vi "Calculate B Matrix.vi"(4 "threshold":dbl=0.0625 format="%#_13g", 6 "Tag ID":i32, 9 "Camera intrinsic matrix (K^-1)":dbl[][](array[numeric]), 10 "Homography H":T1) -> (0 "t (Translation Vector)":dbl[](array[numeric]), 1 "R Rotation Matrix (final)":T1 format="%#_6f", 2 "B Matrix":dbl[][](array[numeric]))   [LabVIEW 2025]
doc: "This VI calculates the full 6-DOF pose of an AprilTag relative to the camera. The algorithm converts the detected homography into camera coordinates using the intrinsic calibration matrix, then computes the tag translation vector and rotation matrix. A predictive filter is applied to the translation vector to reduce jitter and reject outlier measurements."
uses:
  <vilib>/Analysis/Matrix/Datatypes/RealMatrix.ctl
  <vilib>/Analysis/baseanly.llb/Real A x B.vi
  <vilib>/Analysis/baseanly.llb/Real Determinant.vi
  <vilib>/Analysis/7linalg.llb/Real SVD Decomposition.vi
  <vilib>/Analysis/NI_AALPro.lvlib
  <vilib>/Analysis/NI_AALBase.lvlib
  <vilib>/Analysis/Matrix/NI_Matrix.lvlib
panel:
  out "Matrix V":T1
  out "detR":dbl format="%.6f"
  out "detR_temp":dbl format="%.6f"
  out "R^tR":T1 format="%#.3f"
  out "v^t":T1 format="%#_6f"
  out "b1 lambda":dbl
  out "R Matrix":dbl[][](array[numeric])
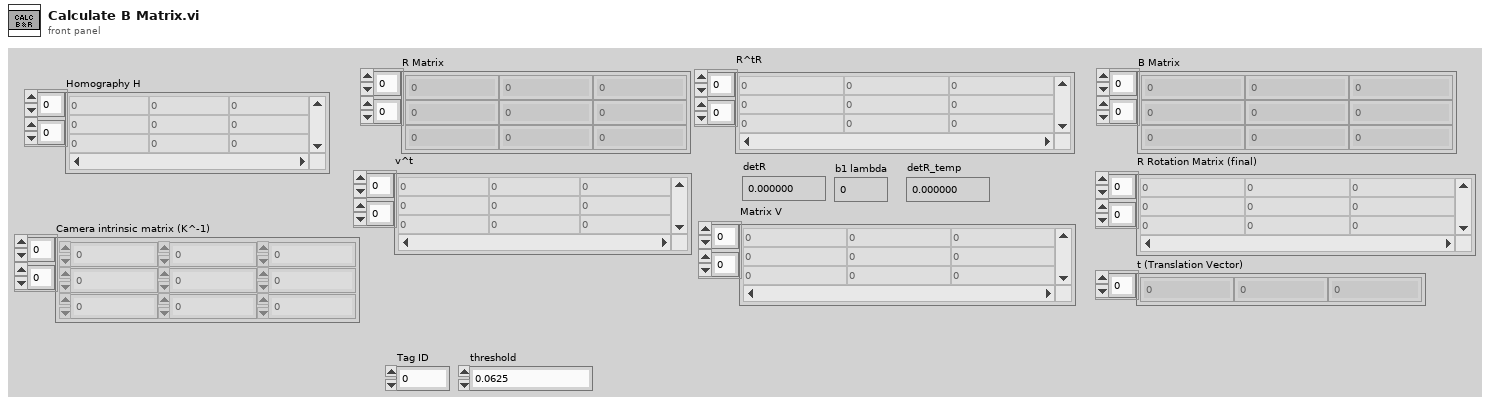
[diagram p1: front panel]
types:
  T1 = typedef "NI_Matrix.lvlib/RealMatrix.ctl" = dbl[][]
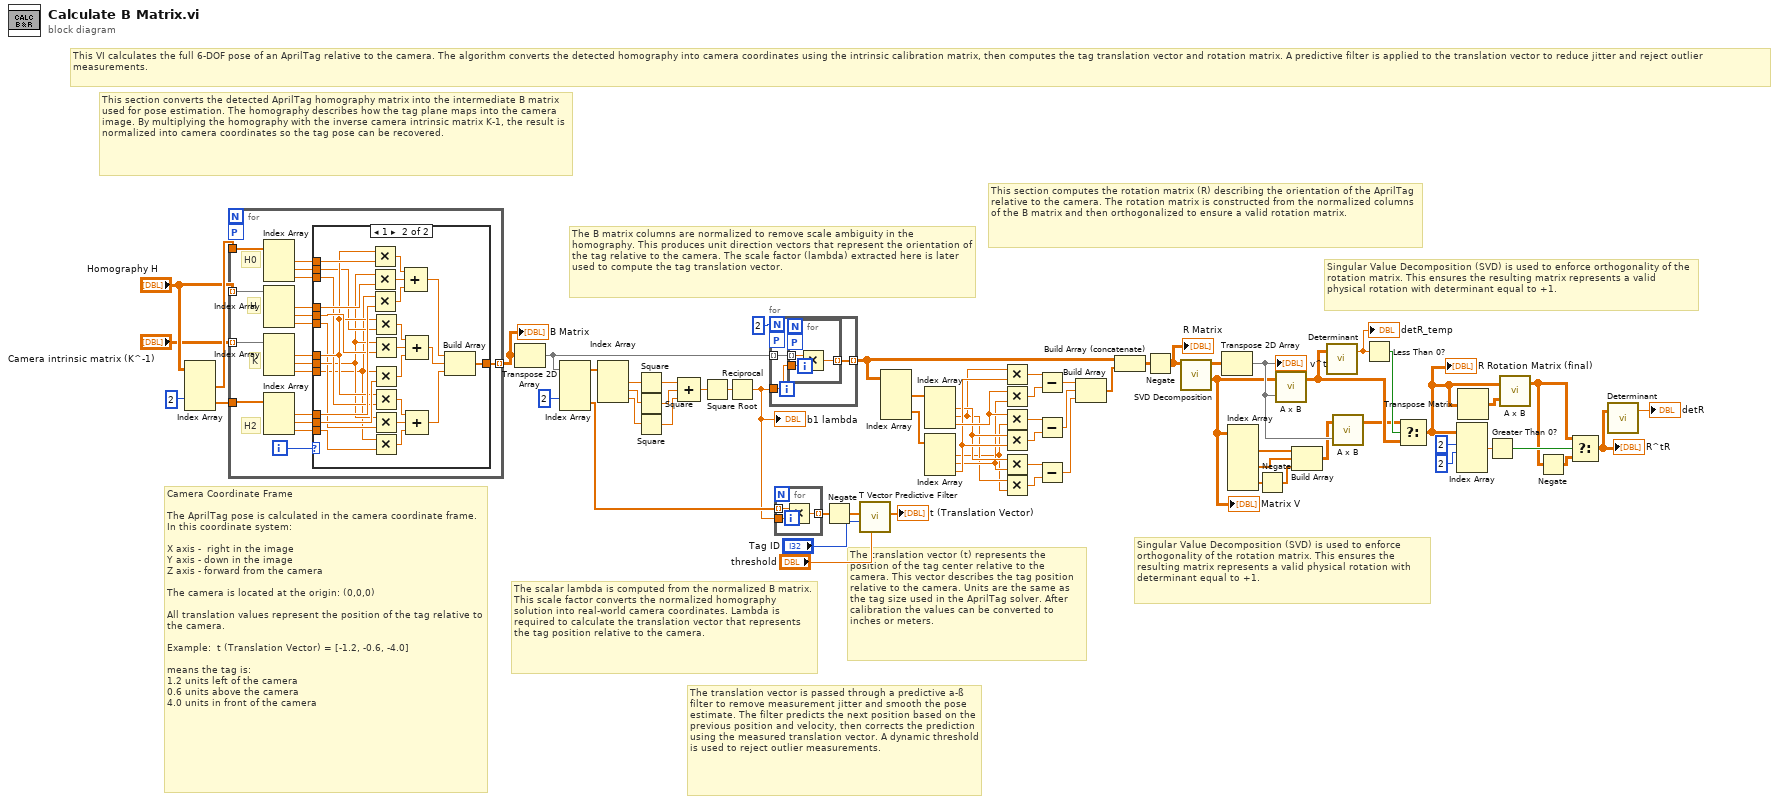
[diagram p0: block diagram]
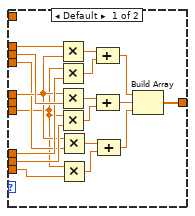
[diagram p2: hidden frame]
diagram:
  # "Camera Coordinate Frame\n\nThe AprilTag pose is calculated in the camera coordinate frame. In this coordinate system:\n\nX axis -  right in the image\nY axis - down in the image\nZ axis - forward from the camera\n\nThe camera is located at the origin: (0,0,0)\n\nAll translation values represent the position of the tag relative to the camera.\n\nExample:  t (Translation Vector) = [-1.2, -0.6, -4.0]\n\nmeans the tag is:\n1.2 units left of the camera\n0.6 units above the camera\n4.0 units in front of the camera"
  # "The translation vector (t) represents the position of the tag center relative to the camera. This vector describes the tag position relative to the camera. Units are the same as the tag size used in the AprilTag solver. After calibration the values can be converted to inches or meters."
  # "This VI calculates the full 6-DOF pose of an AprilTag relative to the camera. The algorithm converts the detected homography into camera coordinates using the intrinsic calibration matrix, then computes the tag translation vector and rotation matrix. A predictive filter is applied to the translation vector to reduce jitter and reject outlier measurements."
  # "Singular Value Decomposition (SVD) is used to enforce orthogonality of the rotation matrix. This ensures the resulting matrix represents a valid physical rotation with determinant equal to +1."
  # "Singular Value Decomposition (SVD) is used to enforce orthogonality of the rotation matrix. This ensures the resulting matrix represents a valid physical rotation with determinant equal to +1."
  # "This section computes the rotation matrix (R) describing the orientation of the AprilTag relative to the camera. The rotation matrix is constructed from the normalized columns of the B matrix and then orthogonalized to ensure a valid rotation matrix."
  # "The scalar lambda is computed from the normalized B matrix. This scale factor converts the normalized homography solution into real-world camera coordinates. Lambda is required to calculate the translation vector that represents the tag position relative to the camera."
  # "The B matrix columns are normalized to remove scale ambiguity in the homography. This produces unit direction vectors that represent the orientation of the tag relative to the camera. The scale factor (lambda) extracted here is later used to compute the tag translation vector."
  # "This section converts the detected AprilTag homography matrix into the intermediate B matrix used for pose estimation. The homography describes how the tag plane maps into the camera image. By multiplying the homography with the inverse camera intrinsic matrix K-1, the result is normalized into camera coordinates so the tag pose can be recovered."
  # "The translation vector is passed through a predictive a-ß filter to remove measurement jitter and smooth the pose estimate. The filter predicts the next position based on the previous position and velocity, then corrects the prediction using the measured translation vector. A dynamic threshold is used to reject outlier measurements."
  n1 = Index Array(array="Homography H", index (row) #2=2 ("index (row)")) -> (element #1=w68:dbl[], element #2=w67:dbl[])  [unwired: 3 in]
  n2 = for {
    tunnel: "Homography H" -> [w85] mode=indexing
    tunnel: "Camera intrinsic matrix (K^-1)" -> [w86] mode=indexing
    tunnel: w67 -> [w82]
    tunnel: [w75] -> w63 mode=indexing
    tunnel: w68 -> [w72]
    workers-P: _ -> [_]
    i -> [w74]
    # "H0"
    # "H2"
    # "K"
    # "H"
    n3 = Index Array(array=w72) -> (element #1=w71:dbl, element #2=w70:dbl, element #3=w69:dbl)  [unwired: 3 in]
    n4 = Index Array(array=w85) -> (element #1=w84:dbl, element #2=w83:dbl, element #3=w78:dbl)  [unwired: 3 in]
    n5 = Index Array(array=w86) -> (element #1=w79:dbl, element #2=w73:dbl, element #3=w77:dbl)  [unwired: 3 in]
    n6 = Index Array(array=w82) -> (element #1=w81:dbl, element #2=w80:dbl, element #3=w76:dbl)  [unwired: 3 in]
    n7 = case shown="1" w74 {
      tunnel: w84 -> [w100 w126]
      tunnel: w83 -> [w99 w118]
      tunnel: w81 -> [w98 w124]
      tunnel: w80 -> [w97 w116]
      tunnel: w79 -> [w94 w112]
      tunnel: w78 -> [w93 w107]
      tunnel: w77 -> [w92 w106]
      tunnel: w76 -> [w91 w105]
      tunnel: [w87 w129] -> w75
      tunnel: w73 -> [_ w108]
      tunnel: w71 -> [_ w128]
      tunnel: w70 -> [_ w111]
      tunnel: w69 -> [_ w109]
      frame Default {
        n8 = Multiply(x=w100, y=w94) -> (x*y=w104:dbl)
        n9 = Multiply(x=w92, y=w98) -> (x*y=w103:dbl)
        n10 = Multiply(x=w94, y=w99) -> (x*y=w102:dbl)
        n11 = Multiply(x=w92, y=w97) -> (x*y=w101:dbl)
        n12 = Multiply(x=w94, y=w93) -> (x*y=w95:dbl)
        n13 = Multiply(x=w92, y=w91) -> (x*y=w96:dbl)
        n14 = Compound Arithmetic op=ADD(w104, w103) -> (w90:dbl)
        n15 = Compound Arithmetic op=ADD(w102, w101) -> (w89:dbl)
        n16 = Compound Arithmetic op=ADD(w95, w96) -> (w88:dbl)
        n17 = Build Array(w90, w89, w88) -> (w87:dbl[])
      }
      frame 1 {
        n18 = Multiply(x=w112, y=w128) -> (x*y=w127:dbl)
        n19 = Multiply(x=w108, y=w126) -> (x*y=w125:dbl)
        n20 = Multiply(x=w106, y=w124) -> (x*y=w123:dbl)
        n21 = Multiply(x=w112, y=w111) -> (x*y=w119:dbl)
        n22 = Multiply(x=w108, y=w118) -> (x*y=w120:dbl)
        n23 = Multiply(x=w106, y=w116) -> (x*y=w121:dbl)
        n24 = Multiply(x=w112, y=w109) -> (x*y=w115:dbl)
        n25 = Multiply(x=w108, y=w107) -> (x*y=w114:dbl)
        n26 = Multiply(x=w106, y=w105) -> (x*y=w113:dbl)
        n27 = Compound Arithmetic op=ADD(w127, w125, w123) -> (w122:dbl)
        n28 = Compound Arithmetic op=ADD(w119, w120, w121) -> (w117:dbl)
        n29 = Compound Arithmetic op=ADD(w115, w114, w113) -> (w110:dbl)
        n30 = Build Array(w122, w117, w110) -> (w129:dbl[])
      }
    }
  }
  "B Matrix" <- w63
  n31 = Transpose 2D Array(2D array=w63) -> (transposed array=w1:dbl[][])
  n32 = Index Array(array=w1, index (row) #2=2 ("index (row)")) -> (element #1=w4:dbl[], element #2=w34:dbl[])  [unwired: 3 in]
  n33 = Index Array(array=w4) -> (element #1=w61:dbl, element #2=w60:dbl, element #3=w59:dbl)  [unwired: 3 in]
  n34 = Square(x=w61) -> (x^2=w58:dbl)
  n35 = Square(x=w60) -> (x^2=w57:dbl)
  n36 = Square(x=w59) -> (x^2=w56:dbl)
  n37 = Compound Arithmetic op=ADD(w58, w57, w56) -> (w55:dbl)
  n38 = Square Root(x=w55) -> (sqrt(x)=w3:dbl)
  n39 = Reciprocal(x=w3) -> (1/x=w2:dbl)
  "b1 lambda" <- w2
  n40 = for {
    N: 2 -> [_]
    tunnel: w1 -> [w132] mode=indexing
    tunnel: w2 -> [w131]
    tunnel: [w130] -> w54 mode=indexing
    workers-P: _ -> [_]
    n41 = for {
      tunnel: w132 -> [w135] mode=indexing
      tunnel: w131 -> [w134]
      tunnel: [w133] -> w130 mode=indexing
      workers-P: _ -> [_]
      n42 = Multiply(x=w135, y=w134) -> (x*y=w133:dbl)
    }
  }
  n43 = for {
    tunnel: w34 -> [w137] mode=indexing
    tunnel: w2 -> [w138]
    tunnel: [w136] -> w33 mode=indexing
    n44 = Multiply(x=w137, y=w138) -> (x*y=w136:dbl)
  }
  n45 = Negate(x=w33) -> (-x=w8:dbl[])
  n46 = call "T Vector Predictive Filter.vi"("threshold"="threshold", "Tag ID"="Tag ID", "t Translation Vector"=w8) -> ("t Translation Vector Prodictive filtered"=→"t (Translation Vector)":dbl[])  [unwired: 8 in]
  n47 = Index Array(array=w54) -> (element #1=w53:dbl[], element #2=w52:dbl[])  [unwired: 4 in]
  n48 = Index Array(array=w53) -> (element #1=w43:dbl, element #2=w41:dbl, element #3=w47:dbl)  [unwired: 3 in]
  n49 = Index Array(array=w52) -> (element #1=w40:dbl, element #2=w42:dbl, element #3=w46:dbl)  [unwired: 3 in]
  n50 = Multiply(x=w41, y=w46) -> (x*y=w51:dbl)
  n51 = Multiply(x=w47, y=w42) -> (x*y=w50:dbl)
  n52 = Multiply(x=w47, y=w40) -> (x*y=w48:dbl)
  n53 = Multiply(x=w43, y=w46) -> (x*y=w49:dbl)
  n54 = Multiply(x=w43, y=w42) -> (x*y=w44:dbl)
  n55 = Multiply(x=w41, y=w40) -> (x*y=w45:dbl)
  n56 = Subtract(x=w51, y=w50) -> (x-y=w39:dbl)
  n57 = Subtract(x=w48, y=w49) -> (x-y=w38:dbl)
  n58 = Subtract(x=w44, y=w45) -> (x-y=w37:dbl)
  n59 = Build Array(w39, w38, w37) -> (w36:dbl[])
  n60 = Build Array (concatenate)(w54, w36) -> (w31:dbl[][])
  n61 = Negate(x=w31) -> (-x=w29:dbl[][])
  "R Matrix" <- w29
  n62 = call-poly <vilib>:"SVD Decomposition.vi"("A"=w29) -> ("Matrix V"=w11:T1, "Matrix U"=w32:T1)  [unwired: 6 in, 3 out]
  "Matrix V" <- w11
  n63 = Transpose 2D Array(2D array=w32) -> (transposed array=w21:T1)
  "v^t" <- w21
  n64 = Index Array(array=w11) -> (element #1=w15:dbl[], element #2=w14:dbl[], element #3=w13:dbl[])  [unwired: 6 in]
  n65 = Negate(x=w13) -> (-x=w12:dbl[])
  n66 = call-poly <vilib>:"A x B.vi"("B"=w21, "A"=w11) -> ("A x B"=w19:T1)  [unwired: 1 out]
  n67 = Build Array(w15, w14, w12) -> (w10:dbl[][])
  n68 = call-poly <vilib>:"Determinant.vi"("Input Matrix"=w19) -> ("determinant"=w22:dbl)  [unwired: 1 in, 1 out]
  "detR_temp" <- w22
  n69 = call-poly <vilib>:"A x B.vi"("B"=w21, "A"=w10) -> ("A x B"=w9:T1)  [unwired: 1 out]
  n70 = Less Than 0?(x=w22) -> (x < 0?=w20:bool)
  n71 = Select(t=w9, s=w20, f=w19) -> (s? t:f=w18:T1)
  "R Rotation Matrix (final)" <- w18
  n72 = Index Array(array=w18, index (row) #1=2 ("index (row)"), index (col) #1=2 ("disabled index (col)")) -> (element #1=w26:dbl)  [unwired: 2 in, 1 out]
  n73 = Transpose Matrix(1:w18) -> (0:w30:T1)
  n74 = Greater Than 0?(x=w26) -> (x > 0?=w25:bool)
  n75 = call-poly <vilib>:"A x B.vi"("B"=w30, "A"=w18) -> ("A x B"=w24:T1)  [unwired: 1 out]
  n76 = Negate(x=w24) -> (-x=w23:T1)
  n77 = Select(t=w24, s=w25, f=w23) -> (s? t:f=w16:T1)
  "R^tR" <- w16
  n78 = call-poly <vilib>:"Determinant.vi"("Input Matrix"=w16) -> ("determinant"=→"detR":dbl)  [unwired: 1 in, 1 out]
